vi "Write.vi"(8 "error in":errorcluster, 9 "File Name":string=" Test.txt", 11 "text":string) -> (0 "error out":errorcluster)   [LabVIEW 2020]
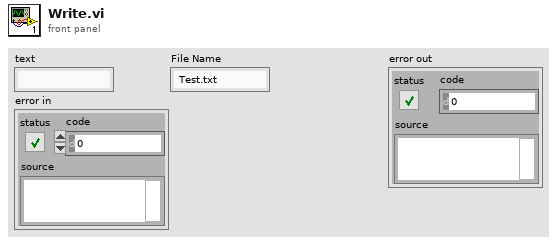
[diagram p1: front panel]
types:
  T1 = enum16{"open", "replace", "create", "open or create", "replace or create", "replace or create with confirmation"}
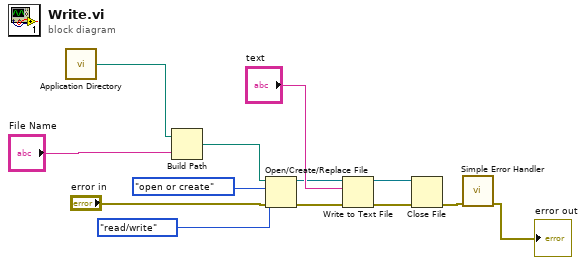
[diagram p0: block diagram]
diagram:
  n1 = call <vilib>:"Application Directory.vi"() -> ("Application Directory"=w2:path)
  n2 = Build Path(base path=w2, name or relative path="File Name") -> (appended path=w6:path)
  n3 = Open/Create/Replace File(file path (use dialog)=w6, error in="error in", operation (0:open)=T1."open or create", access (0:read/write)=enum16{"read/write", "read-only", "write-only"}."read/write") -> (refnum out=w5:refnum<file>, error out=w10:errorcluster)  [unwired: 2 in, 1 out]
  n4 = Write to Text File(file (use dialog)=w5, text="text", error in=w10) -> (refnum out=w9:refnum<file>, error out=w8:errorcluster)  [unwired: 1 in, 1 out]
  n5 = Close File(refnum=w9, error in=w8) -> (error out=w4:errorcluster)  [unwired: 1 out]
  n6 = call <vilib>:"Simple Error Handler.vi"("error in (no error)"=w4) -> ("error out"=→"error out":errorcluster)  [unwired: 4 in, 4 out]
